vi "全局变量1.vi"() -> ()   [LabVIEW 2016, in "TCP文件传输系统.lvlib"]
panel:
  out "TCP接收全局簇":T1={"网络灯"=FALSE, "接收中"=TRUE, "已接收百分比"="", "接收成功次数"=0.0}
  out "TCP发送全局簇":T2={"网络灯"=FALSE, "发送中"=TRUE, "已发送百分比"="", "发送成功次数"=0.0}
  out "传输次数":dbl
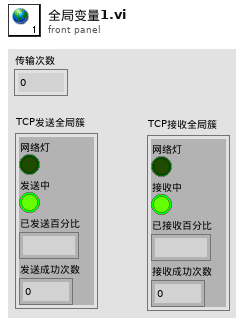
[diagram p1: front panel]
types:
  T1 = cluster{"网络灯":bool, "接收中":bool, "已接收百分比":string, "接收成功次数":dbl}
  T2 = cluster{"网络灯":bool, "发送中":bool, "已发送百分比":string, "发送成功次数":dbl}
diagram:
